vi "Prepare Numeric Patterns.vi"() -> (3 "Numeric Patterns":T1[](array[typedef]))   [LabVIEW 2011, in "Super Simple Neural Network.lvlib"]
uses:
  Super Simple Neural Network.lvlib
  Types/1D Array.ctl
  Types/Teaching Vector.ctl
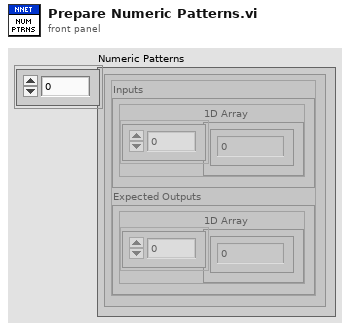
[diagram p1: front panel]
types:
  T1 = typedef "Super Simple Neural Network.lvlib/Teaching Vector.ctl" = cluster{"Inputs":T2, "Expected Outputs":T2}
  T2 = typedef "Super Simple Neural Network.lvlib/1D Array.ctl" = cluster{"1D Array":dbl[]}
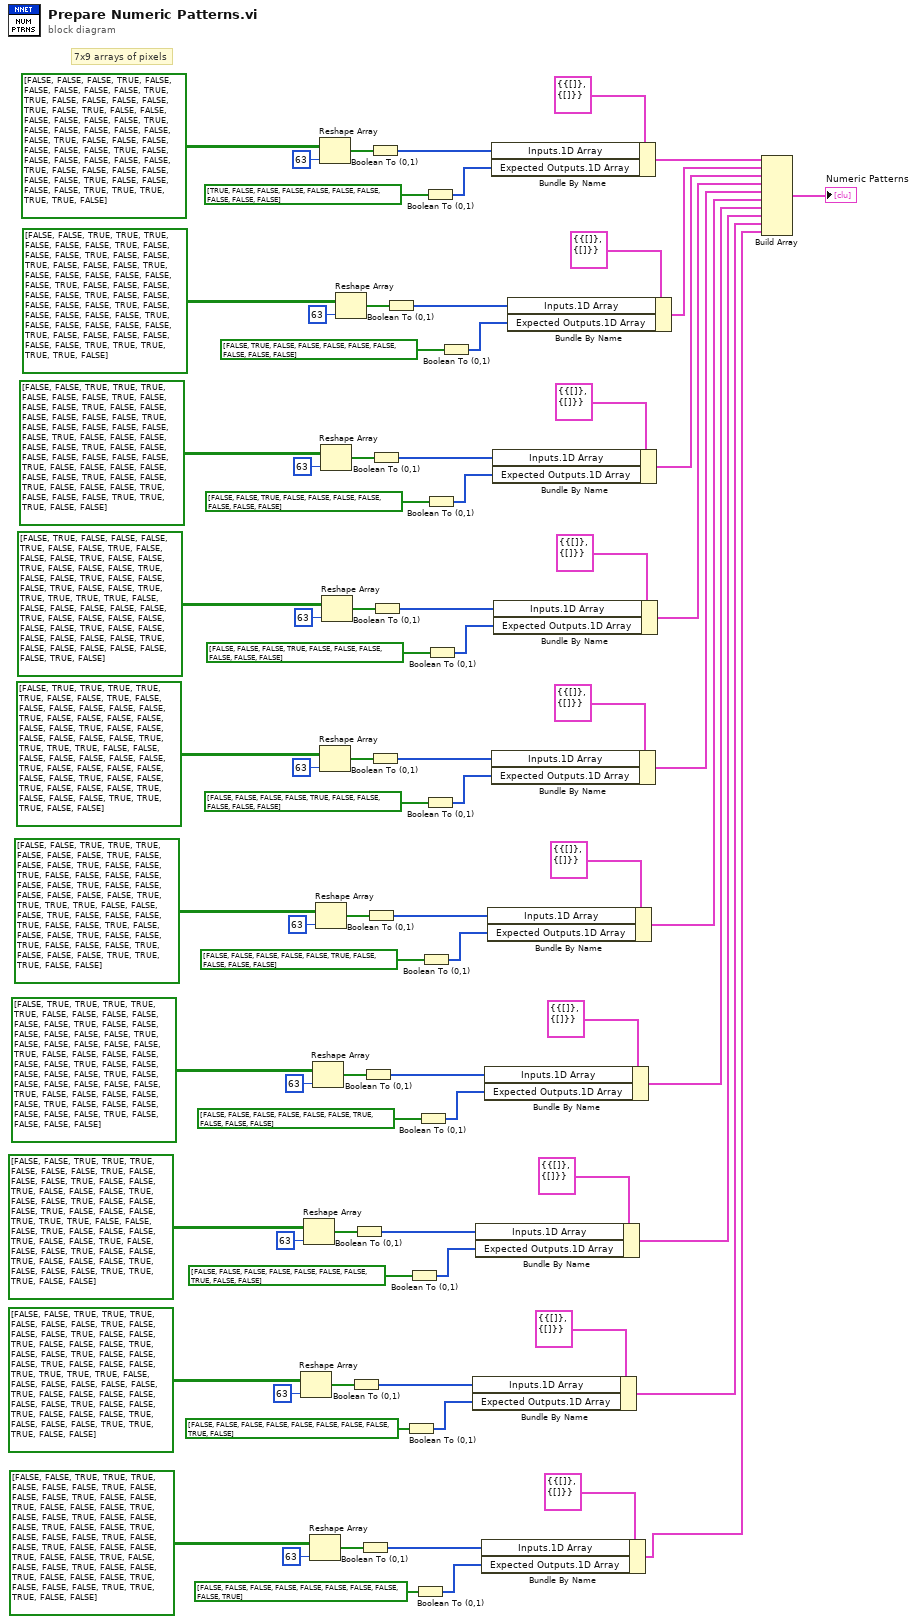
[diagram p0: block diagram]
diagram:
  # "7x9 arrays of pixels"
  n1 = Reshape Array(bool[][] [[FALSE, FALSE, TRUE, TRUE, TRUE, FALSE, FALSE], [FALSE, TRUE, FALSE, FALSE, FALSE, TRUE, FALSE], [FALSE, TRUE, FALSE, FALSE, FALSE, TRUE, FALSE], [FALSE, TRUE, FALSE, FALSE, FALSE, TRUE, FALSE], [FALSE, FALSE, TRUE, TRUE, TRUE, TRUE, FALSE], [FALSE, FALSE, FALSE, FALSE, FALSE, TRUE, FALSE], [FALSE, FALSE, FALSE, FALSE, FALSE, TRUE, FALSE], [FALSE, TRUE, FALSE, FALSE, FALSE, TRUE, FALSE], [FALSE, FALSE, TRUE, TRUE, TRUE, FALSE, FALSE]] ("Pixels Pattern"), 63 ("dimension size")) -> (w52:bool[])
  n2 = Reshape Array(bool[][] [[FALSE, FALSE, TRUE, TRUE, TRUE, FALSE, FALSE], [FALSE, TRUE, FALSE, FALSE, FALSE, TRUE, FALSE], [FALSE, TRUE, FALSE, FALSE, FALSE, TRUE, FALSE], [FALSE, TRUE, FALSE, FALSE, FALSE, TRUE, FALSE], [FALSE, FALSE, TRUE, TRUE, TRUE, FALSE, FALSE], [FALSE, TRUE, FALSE, FALSE, FALSE, TRUE, FALSE], [FALSE, TRUE, FALSE, FALSE, FALSE, TRUE, FALSE], [FALSE, TRUE, FALSE, FALSE, FALSE, TRUE, FALSE], [FALSE, FALSE, TRUE, TRUE, TRUE, FALSE, FALSE]] ("Pixels Pattern"), 63 ("dimension size")) -> (w49:bool[])
  n3 = Reshape Array(bool[][] [[FALSE, FALSE, TRUE, TRUE, TRUE, FALSE, FALSE], [FALSE, TRUE, FALSE, FALSE, FALSE, TRUE, FALSE], [FALSE, TRUE, FALSE, FALSE, FALSE, TRUE, FALSE], [FALSE, TRUE, FALSE, FALSE, FALSE, TRUE, FALSE], [FALSE, TRUE, FALSE, FALSE, FALSE, TRUE, FALSE], [FALSE, TRUE, FALSE, FALSE, FALSE, TRUE, FALSE], [FALSE, TRUE, FALSE, FALSE, FALSE, TRUE, FALSE], [FALSE, TRUE, FALSE, FALSE, FALSE, TRUE, FALSE], [FALSE, FALSE, TRUE, TRUE, TRUE, FALSE, FALSE]] ("Pixels Pattern"), 63 ("dimension size")) -> (w61:bool[])
  n4 = Reshape Array(bool[][] [[FALSE, TRUE, TRUE, TRUE, TRUE, TRUE, FALSE], [FALSE, FALSE, FALSE, FALSE, FALSE, TRUE, FALSE], [FALSE, FALSE, FALSE, FALSE, FALSE, TRUE, FALSE], [FALSE, FALSE, FALSE, FALSE, TRUE, FALSE, FALSE], [FALSE, FALSE, FALSE, FALSE, TRUE, FALSE, FALSE], [FALSE, FALSE, FALSE, TRUE, FALSE, FALSE, FALSE], [FALSE, FALSE, FALSE, TRUE, FALSE, FALSE, FALSE], [FALSE, FALSE, TRUE, FALSE, FALSE, FALSE, FALSE], [FALSE, FALSE, TRUE, FALSE, FALSE, FALSE, FALSE]] ("Pixels Pattern"), 63 ("dimension size")) -> (w40:bool[])
  n5 = Reshape Array(bool[][] [[FALSE, FALSE, TRUE, TRUE, TRUE, FALSE, FALSE], [FALSE, TRUE, FALSE, FALSE, FALSE, TRUE, FALSE], [FALSE, TRUE, FALSE, FALSE, FALSE, FALSE, FALSE], [FALSE, TRUE, FALSE, FALSE, FALSE, FALSE, FALSE], [FALSE, TRUE, TRUE, TRUE, TRUE, FALSE, FALSE], [FALSE, TRUE, FALSE, FALSE, FALSE, TRUE, FALSE], [FALSE, TRUE, FALSE, FALSE, FALSE, TRUE, FALSE], [FALSE, TRUE, FALSE, FALSE, FALSE, TRUE, FALSE], [FALSE, FALSE, TRUE, TRUE, TRUE, FALSE, FALSE]] ("Pixels Pattern"), 63 ("dimension size")) -> (w37:bool[])
  n6 = Reshape Array(bool[][] [[FALSE, FALSE, FALSE, TRUE, FALSE, FALSE, FALSE], [FALSE, FALSE, TRUE, TRUE, FALSE, FALSE, FALSE], [FALSE, TRUE, FALSE, TRUE, FALSE, FALSE, FALSE], [FALSE, FALSE, FALSE, TRUE, FALSE, FALSE, FALSE], [FALSE, FALSE, FALSE, TRUE, FALSE, FALSE, FALSE], [FALSE, FALSE, FALSE, TRUE, FALSE, FALSE, FALSE], [FALSE, FALSE, FALSE, TRUE, FALSE, FALSE, FALSE], [FALSE, FALSE, FALSE, TRUE, FALSE, FALSE, FALSE], [FALSE, TRUE, TRUE, TRUE, TRUE, TRUE, FALSE]] ("Pixels Pattern"), 63 ("dimension size")) -> (w3:bool[])
  n7 = Reshape Array(bool[][] [[FALSE, TRUE, TRUE, TRUE, TRUE, TRUE, FALSE], [FALSE, TRUE, FALSE, FALSE, FALSE, FALSE, FALSE], [FALSE, TRUE, FALSE, FALSE, FALSE, FALSE, FALSE], [FALSE, TRUE, FALSE, FALSE, FALSE, FALSE, FALSE], [FALSE, TRUE, TRUE, TRUE, TRUE, FALSE, FALSE], [FALSE, FALSE, FALSE, FALSE, FALSE, TRUE, FALSE], [FALSE, FALSE, FALSE, FALSE, FALSE, TRUE, FALSE], [FALSE, TRUE, FALSE, FALSE, FALSE, TRUE, FALSE], [FALSE, FALSE, TRUE, TRUE, TRUE, FALSE, FALSE]] ("Pixels Pattern"), 63 ("dimension size")) -> (w28:bool[])
  n8 = Reshape Array(bool[][] [[FALSE, FALSE, TRUE, TRUE, TRUE, FALSE, FALSE], [FALSE, TRUE, FALSE, FALSE, FALSE, TRUE, FALSE], [FALSE, FALSE, FALSE, FALSE, FALSE, TRUE, FALSE], [FALSE, FALSE, FALSE, FALSE, FALSE, TRUE, FALSE], [FALSE, FALSE, FALSE, FALSE, TRUE, FALSE, FALSE], [FALSE, FALSE, FALSE, FALSE, FALSE, TRUE, FALSE], [FALSE, FALSE, FALSE, FALSE, FALSE, TRUE, FALSE], [FALSE, TRUE, FALSE, FALSE, FALSE, TRUE, FALSE], [FALSE, FALSE, TRUE, TRUE, TRUE, FALSE, FALSE]] ("Pixels Pattern"), 63 ("dimension size")) -> (w16:bool[])
  n9 = Reshape Array(bool[][] [[FALSE, TRUE, FALSE, FALSE, FALSE, TRUE, FALSE], [FALSE, TRUE, FALSE, FALSE, FALSE, TRUE, FALSE], [FALSE, TRUE, FALSE, FALSE, FALSE, TRUE, FALSE], [FALSE, TRUE, FALSE, FALSE, FALSE, TRUE, FALSE], [FALSE, TRUE, TRUE, TRUE, TRUE, TRUE, FALSE], [FALSE, FALSE, FALSE, FALSE, FALSE, TRUE, FALSE], [FALSE, FALSE, FALSE, FALSE, FALSE, TRUE, FALSE], [FALSE, FALSE, FALSE, FALSE, FALSE, TRUE, FALSE], [FALSE, FALSE, FALSE, FALSE, FALSE, TRUE, FALSE]] ("Pixels Pattern"), 63 ("dimension size")) -> (w25:bool[])
  n10 = Reshape Array(bool[][] [[FALSE, FALSE, TRUE, TRUE, TRUE, FALSE, FALSE], [FALSE, TRUE, FALSE, FALSE, FALSE, TRUE, FALSE], [FALSE, TRUE, FALSE, FALSE, FALSE, TRUE, FALSE], [FALSE, FALSE, FALSE, FALSE, FALSE, TRUE, FALSE], [FALSE, FALSE, FALSE, FALSE, TRUE, FALSE, FALSE], [FALSE, FALSE, FALSE, TRUE, FALSE, FALSE, FALSE], [FALSE, FALSE, TRUE, FALSE, FALSE, FALSE, FALSE], [FALSE, TRUE, FALSE, FALSE, FALSE, FALSE, FALSE], [FALSE, TRUE, TRUE, TRUE, TRUE, TRUE, FALSE]] ("Pixels Pattern"), 63 ("dimension size")) -> (w12:bool[])
  n11 = Boolean To (0,1)(Boolean=w52) -> (0, 1=w53:i16[])
  n12 = Boolean To (0,1)(Boolean=w49) -> (0, 1=w48:i16[])
  n13 = Boolean To (0,1)(Boolean=w61) -> (0, 1=w60:i16[])
  n14 = Boolean To (0,1)(Boolean=w40) -> (0, 1=w41:i16[])
  n15 = Boolean To (0,1)(Boolean=w37) -> (0, 1=w36:i16[])
  n16 = Boolean To (0,1)(Boolean=w3) -> (0, 1=w4:i16[])
  n17 = Boolean To (0,1)(Boolean=w28) -> (0, 1=w29:i16[])
  n18 = Boolean To (0,1)(Boolean=w16) -> (0, 1=w17:i16[])
  n19 = Boolean To (0,1)(Boolean=w25) -> (0, 1=w24:i16[])
  n20 = Boolean To (0,1)(Boolean=w12) -> (0, 1=w11:i16[])
  n21 = Boolean To (0,1)(Boolean=bool[] [FALSE, FALSE, FALSE, FALSE, FALSE, FALSE, FALSE, FALSE, TRUE, FALSE] ("output array")) -> (0, 1=w56:i16[])
  n22 = Boolean To (0,1)(Boolean=bool[] [FALSE, FALSE, FALSE, FALSE, FALSE, FALSE, FALSE, TRUE, FALSE, FALSE] ("output array")) -> (0, 1=w45:i16[])
  n23 = Boolean To (0,1)(Boolean=bool[] [FALSE, FALSE, FALSE, FALSE, FALSE, FALSE, FALSE, FALSE, FALSE, TRUE] ("output array")) -> (0, 1=w57:i16[])
  n24 = Boolean To (0,1)(Boolean=bool[] [FALSE, FALSE, FALSE, FALSE, FALSE, FALSE, TRUE, FALSE, FALSE, FALSE] ("output array")) -> (0, 1=w44:i16[])
  n25 = Boolean To (0,1)(Boolean=bool[] [FALSE, FALSE, FALSE, FALSE, FALSE, TRUE, FALSE, FALSE, FALSE, FALSE] ("output array")) -> (0, 1=w33:i16[])
  n26 = Boolean To (0,1)(Boolean=bool[] [TRUE, FALSE, FALSE, FALSE, FALSE, FALSE, FALSE, FALSE, FALSE, FALSE] ("output array")) -> (0, 1=w7:i16[])
  n27 = Boolean To (0,1)(Boolean=bool[] [FALSE, FALSE, FALSE, FALSE, TRUE, FALSE, FALSE, FALSE, FALSE, FALSE] ("output array")) -> (0, 1=w32:i16[])
  n28 = Boolean To (0,1)(Boolean=bool[] [FALSE, FALSE, TRUE, FALSE, FALSE, FALSE, FALSE, FALSE, FALSE, FALSE] ("output array")) -> (0, 1=w20:i16[])
  n29 = Boolean To (0,1)(Boolean=bool[] [FALSE, FALSE, FALSE, TRUE, FALSE, FALSE, FALSE, FALSE, FALSE, FALSE] ("output array")) -> (0, 1=w21:i16[])
  n30 = Boolean To (0,1)(Boolean=bool[] [FALSE, TRUE, FALSE, FALSE, FALSE, FALSE, FALSE, FALSE, FALSE, FALSE] ("output array")) -> (0, 1=w8:i16[])
  n31 = Bundle By Name(cluster=T1 {"Inputs"={"1D Array"=[]}, "Expected Outputs"={"1D Array"=[]}} ("Teaching Vector"), "Inputs.1D Array"=w53, "Expected Outputs.1D Array"=w56) -> (w79:T1)
  n32 = Bundle By Name(cluster=T1 {"Inputs"={"1D Array"=[]}, "Expected Outputs"={"1D Array"=[]}} ("Teaching Vector"), "Inputs.1D Array"=w48, "Expected Outputs.1D Array"=w45) -> (w78:T1)
  n33 = Bundle By Name(cluster=T1 {"Inputs"={"1D Array"=[]}, "Expected Outputs"={"1D Array"=[]}} ("Teaching Vector"), "Inputs.1D Array"=w60, "Expected Outputs.1D Array"=w57) -> (w80:T1)
  n34 = Bundle By Name(cluster=T1 {"Inputs"={"1D Array"=[]}, "Expected Outputs"={"1D Array"=[]}} ("Teaching Vector"), "Inputs.1D Array"=w41, "Expected Outputs.1D Array"=w44) -> (w77:T1)
  n35 = Bundle By Name(cluster=T1 {"Inputs"={"1D Array"=[]}, "Expected Outputs"={"1D Array"=[]}} ("Teaching Vector"), "Inputs.1D Array"=w36, "Expected Outputs.1D Array"=w33) -> (w76:T1)
  n36 = Bundle By Name(cluster=T1 {"Inputs"={"1D Array"=[]}, "Expected Outputs"={"1D Array"=[]}} ("Teaching Vector"), "Inputs.1D Array"=w4, "Expected Outputs.1D Array"=w7) -> (w71:T1)
  n37 = Bundle By Name(cluster=T1 {"Inputs"={"1D Array"=[]}, "Expected Outputs"={"1D Array"=[]}} ("Teaching Vector"), "Inputs.1D Array"=w29, "Expected Outputs.1D Array"=w32) -> (w75:T1)
  n38 = Bundle By Name(cluster=T1 {"Inputs"={"1D Array"=[]}, "Expected Outputs"={"1D Array"=[]}} ("Teaching Vector"), "Inputs.1D Array"=w17, "Expected Outputs.1D Array"=w20) -> (w73:T1)
  n39 = Bundle By Name(cluster=T1 {"Inputs"={"1D Array"=[]}, "Expected Outputs"={"1D Array"=[]}} ("Teaching Vector"), "Inputs.1D Array"=w24, "Expected Outputs.1D Array"=w21) -> (w74:T1)
  n40 = Bundle By Name(cluster=T1 {"Inputs"={"1D Array"=[]}, "Expected Outputs"={"1D Array"=[]}} ("Teaching Vector"), "Inputs.1D Array"=w11, "Expected Outputs.1D Array"=w8) -> (w72:T1)
  n41 = Build Array(w71, w72, w73, w74, w75, w76, w77, w78, w79, w80) -> (→"Numeric Patterns":T1[])
